vi "disturbance.vi"(4 "y(k)":dbl[](array[numeric])) -> (1 "ym(k)":dbl[](array[numeric]))   [LabVIEW 2017]
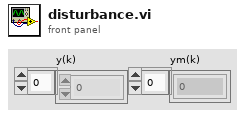
[diagram p1: front panel]
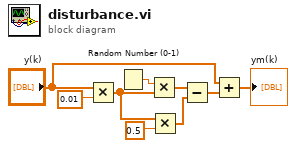
[diagram p0: block diagram]
diagram:
  n1 = Multiply(x="y(k)", y=0.01) -> (x*y=w5:dbl[])
  n2 = Random Number (0-1)() -> (number: 0 to 1=w6:dbl)
  n3 = Multiply(x=w6, y=w5) -> (x*y=w7:dbl[])
  n4 = Multiply(x=w5, y=0.5) -> (x*y=w8:dbl[])
  n5 = Subtract(x=w7, y=w8) -> (x-y=w9:dbl[])
  n6 = Add(x="y(k)", y=w9) -> (x+y=→"ym(k)":dbl[])
